vi "Update Actor List.vi"(8 "Error In":errorcluster, 11 "CS++ObjectManager in":refnum<class "CS++ObjectManager.lvclass">) -> (0 "Error Out":errorcluster, 3 "CS++ObjectManager out":refnum<class "CS++ObjectManager.lvclass">)   [LabVIEW 2014, in "CS++ObjectManager.lvlib" / "CS++ObjectManager.lvclass"]
doc: "Update Actor List from FGV Actor Enqueuer.vi and send to GUI."
uses:
  CS++ObjectManager.lvclass
  CSPP_Core/Libraries/Base/FGV Action.ctl
  CS++ObjectManager.lvclass/CS++ObjectManager.ctl
  CSPP_Core/Libraries/Base/CS++Base.lvlib
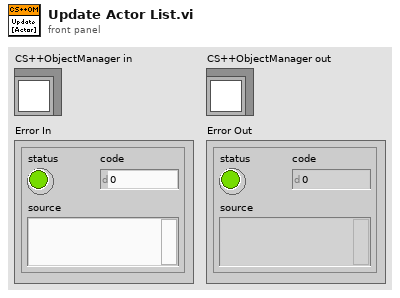
[diagram p1: front panel]
types:
  T1 = typedef "CS++Base.lvlib/FGV Action.ctl" = enum16{"add", "replace", "read", "remove", "reset", "get attributes"}
  T2 = cluster{"Class Name":string, "Enqueuer":refnum<class "Message Enqueuer.lvclass">}[]
  T3 = cluster{"Actor Names":string[], "Actor Class & Enqueuer":cluster{"Class Name":string, "Enqueuer":refnum<class "Message Enqueuer.lvclass">}[]}
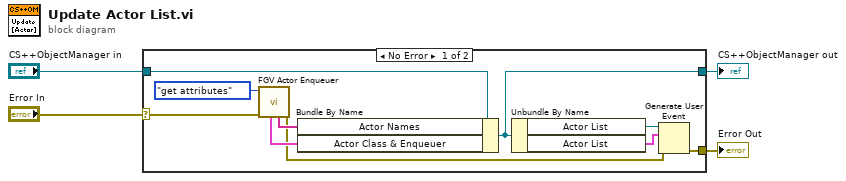
[diagram p0: block diagram]
diagram:
  n1 = case shown="No Error" "Error In" {
    selector: "Error In" -> [w11 w16]
    tunnel: [w5 w16] -> w3
    tunnel: [w9 w15] -> w1
    tunnel: "CS++ObjectManager in" -> [w10 w15]
    frame No Error {
      n2 = call "FGV Actor Enqueuer.vi"("Error In"=w11, "Action (read)"=FGV_Action."get attributes") -> ("Error Out"=w6:errorcluster, "[Actor Name]"=w13:string[], "[Class & Enqueuer]"=w12:T2)  [unwired: 5 in, 2 out]
      n3 = Bundle By Name(cluster=w10, "Actor Names"=w13, "Actor Class & Enqueuer"=w12) -> (w9:refnum<class "CS++ObjectManager.lvclass">)
      n4 = Unbundle By Name(w9) -> ("Actor List"=w8:refnum<user-event>, "Actor List"=w7:T3)
      n5 = Generate User Event(user event=w8, event data cluster=w7, error in=w6) -> (error out=w5:errorcluster)  [unwired: 1 in, 1 out]
    }
    frame Error {
    }
  }
  "Error Out" <- w3
  "CS++ObjectManager out" <- w1
